vi "Perform IMD Measurement.vi"(7 "measurement configuration":T2={"Full scale range"=2.825, "Channel name"="", "Analog source resource name"="", "IMD standard"=enum."SMPTE (60 Hz, 7000 Hz, 4:1)", "Low frequency"=0.0, "High frequency"=0.0, "Amplitude ratio"=0.0, "Amplitude"=0.0, "Protocol capture resource name"="", "Data line"=0, "Channel"=0, "Sample rate"=44100.0, "Measurement duration"=0.1, "Frame sync edge for Channel 0"=enum."Falling", "Channel count per frame"=2, "Channel length"=32, "Bit depth"=24, "Channel 0 offset"=1, "Endianness"=enum."MSB First", "Data Justification"=enum."Left Justified", "Frame length"=64, "Frame sync pulse width"=32, "Bit clock edge  sync"=enum."Falling"}, 8 "error in":errorcluster, 11 "PCM waveforms":waveform(dbl)[](array[waveform])) -> (0 "error out":errorcluster, 3 "measurement results":T1)   [LabVIEW 2021, in "IMD_Audio ADC.lvlib"]
uses:
  IMD_Audio ADC.lvlib
  Measurement Configuration.ctl
  Measurement Results.ctl
  <vilib>/addons/_NISVFA/_Shared subVIs/Common/SVL Set dB Reference (1 Ch).vi
  <vilib>/addons/_NISVFA/_Shared subVIs/Common/SVL Set dB Reference (variant).vi
  <vilib>/addons/_NISVFA/_Shared subVIs/Common/svc_Caller VI Returned in Error Source.vi
  <vilib>/addons/Sound and Vibration/svt_Distortion/SVT Intermodulation Distortion (1 Ch).vi
  <vilib>/addons/Sound and Vibration/svt_Distortion/SoundVib_Distortion.lvlib
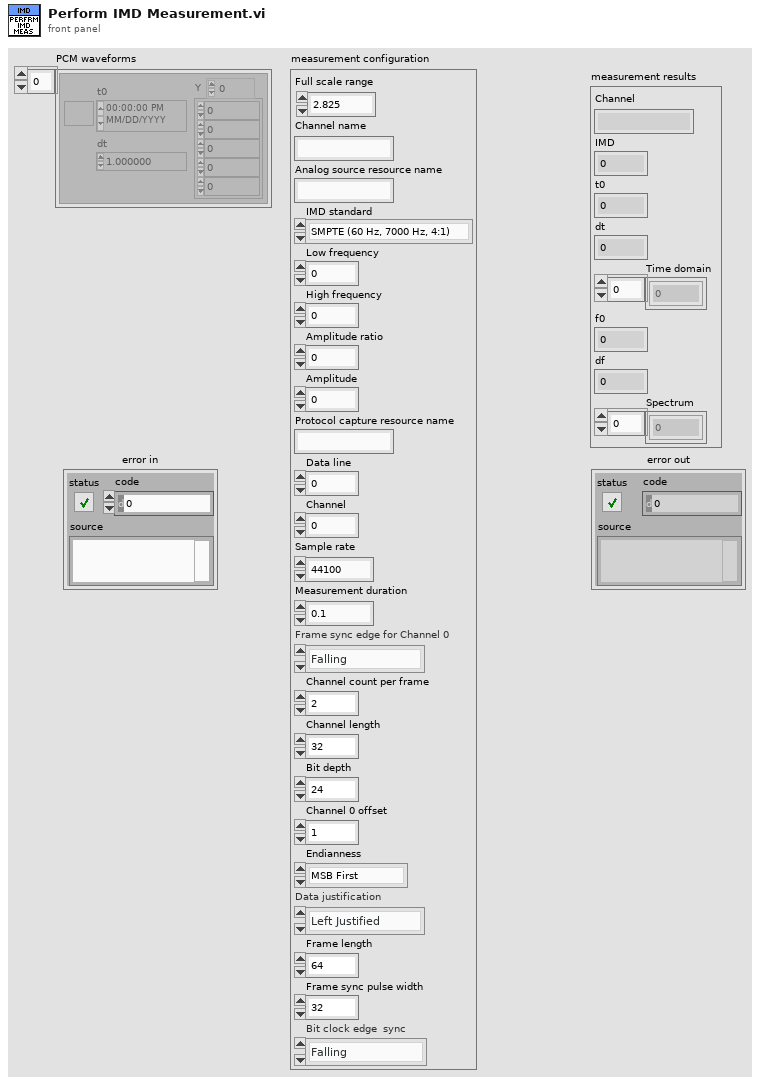
[diagram p1: front panel]
types:
  T1 = typedef "IMD_Audio ADC.lvlib/Measurement Results.ctl" = cluster{"Channel":string, "IMD":dbl, "t0":dbl, "dt":dbl, "Time domain":dbl[], "f0":dbl, "df":dbl, "Spectrum":dbl[]}
  T2 = typedef "IMD_Audio ADC.lvlib/Measurement Configuration.ctl" = cluster{"Full scale range":dbl, "Channel name":string, "Analog source resource name":string, "IMD standard":enum32{"SMPTE (60 Hz, 7000 Hz, 4:1)", "DIN (250 Hz, 8000 Hz, 4:1)", "CCIF (11 kHz, 12 kHz, 1:1)", "CCIF (19 kHz, 20 kHz, 1:1)", "Custom"}, "Low frequency":dbl, "High frequency":dbl, "Amplitude ratio":dbl, "Amplitude":dbl, "Protocol capture resource name":string, "Data line":u32, "Channel":u32, "Sample rate":dbl, "Measurement duration":dbl, "Frame sync edge for Channel 0":enum32{"Rising", "Falling"}, "Channel count per frame":u32, "Channel length":u32, "Bit depth":u32, "Channel 0 offset":u32, "Endianness":enum32{"MSB First", "LSB First"}, "Data Justification":enum32{"Left Justified", "Right Justified"}, "Frame length":u32, "Frame sync pulse width":u32, "Bit clock edge  sync":enum32{"Rising", "Falling"}}
  T3 = cluster{"IMD type":enum16{"SMPTE/DIN", "CCIF/Twin-Tone"}, "low-frequency tone":dbl, "high-frequency tone":dbl, "amplitude ratio":dbl, "maximum order":i32}
  T4 = enum32{"SMPTE (60 Hz, 7000 Hz, 4:1)", "DIN (250 Hz, 8000 Hz, 4:1)", "CCIF (11 kHz, 12 kHz, 1:1)", "CCIF (19 kHz, 20 kHz, 1:1)", "Custom"}
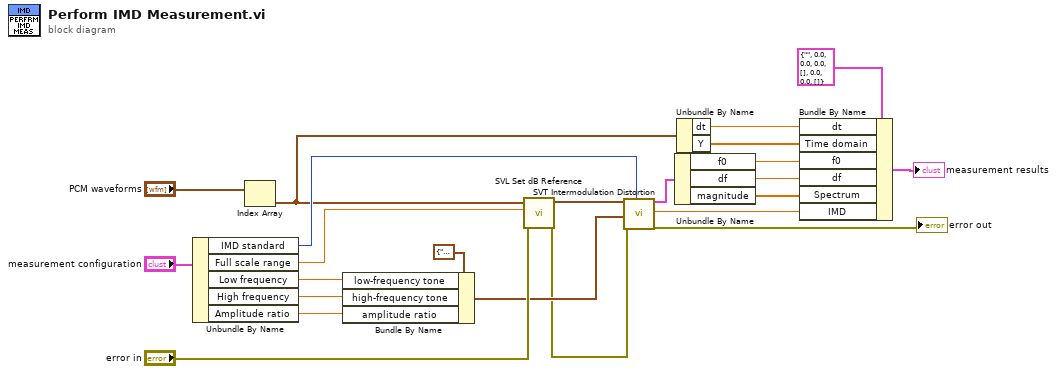
[diagram p0: block diagram]
diagram:
  n1 = Unbundle By Name("measurement configuration") -> ("IMD standard"=w17:T4, "Full scale range"=w18:dbl, "Low frequency"=w22:dbl, "High frequency"=w21:dbl, "Amplitude ratio"=w19:dbl)
  n2 = Index Array(array="PCM waveforms") -> (element=w11:waveform(dbl))  [unwired: 1 in]
  n3 = Bundle By Name(cluster=T3 {"IMD type"=enum."CCIF/Twin-Tone", "low-frequency tone"=14000.0, "high-frequency tone"=15000.0, "amplitude ratio"=1.0, "maximum order"=5} ("custom IMD signal"), "low-frequency tone"=w22, "high-frequency tone"=w21, "amplitude ratio"=w19) -> (w13:T3)
  n4 = call-poly <vilib>:"SVL Set dB Reference.vi"("error in (no error)"="error in", "dB reference [EU]"=w18, "scaled signal in [EU]"=w11) -> ("error out"=w12:errorcluster, "scaled signal out [EU]"=w14:waveform(dbl))  [unwired: 7 in]
  n5 = call-poly <vilib>:"SVT Intermodulation Distortion.vi"("scaled signal [EU]"=w14, "custom IMD signal"=w13, "error in"=w12, "IMD standard"=w17) -> ("magnitude spectrum"=w10:cluster{"f0":dbl, "df":dbl, "magnitude":dbl[]}, "IMD"=w3:dbl, "error out"=→"error out":errorcluster)  [unwired: 8 in, 5 out]
  n6 = Unbundle By Name(w10) -> ("f0"=w6:dbl, "df"=w5:dbl, "magnitude"=w4:dbl[])
  n7 = Unbundle By Name(w11) -> ("dt"=w8:dbl, "Y"=w7:dbl[])
  n8 = Bundle By Name(cluster=T1 {"Channel"="", "IMD"=0.0, "t0"=0.0, "dt"=0.0, "Time domain"=[], "f0"=0.0, "df"=0.0, "Spectrum"=[]} ("measurement results"), "dt"=w8, "Time domain"=w7, "f0"=w6, "df"=w5, "Spectrum"=w4, "IMD"=w3) -> (→"measurement results":T1)
